vi "ConvertFormatElementsToItemList.vi"(11 "Format Elements":T1[](array[typedef])) -> (3 "Item List":string)   [LabVIEW 2012, in "Keithley-6485.lvlib"]
uses:
  Keithley-6485.lvlib
  Public/Controls/FormatElement.ctl
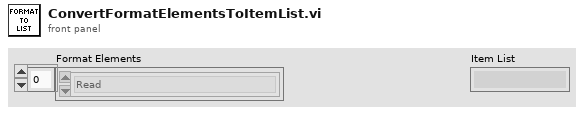
[diagram p1: front panel]
types:
  T1 = typedef "Keithley-6485.lvlib/FormatElement.ctl" = enum16{"Read", "Unit", "Time", "Status"}
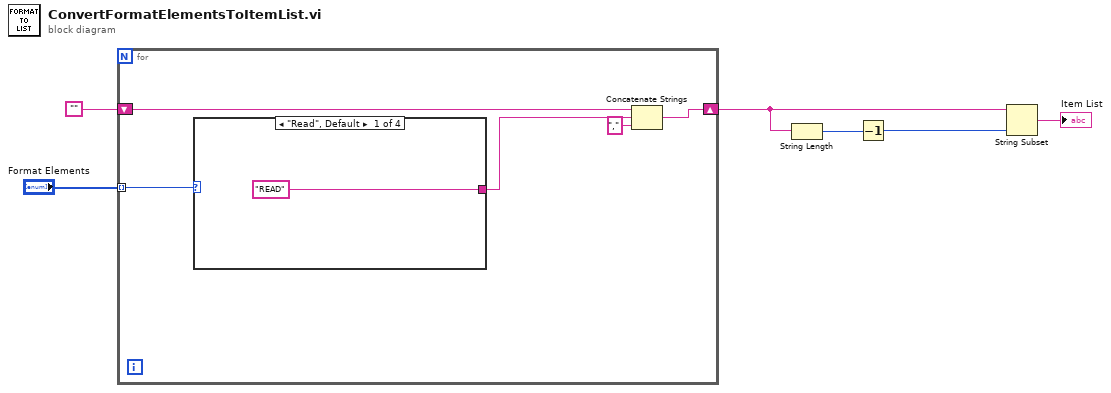
[diagram p0: block diagram]
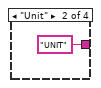
[diagram p2: hidden frame]
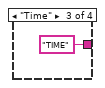
[diagram p3: hidden frame]
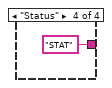
[diagram p4: hidden frame]
diagram:
  n1 = for {
    tunnel: "Format Elements" -> [w9] mode=indexing
    shift-right: [w10] -> w4
    shift-left: "" -> [w11]
    n2 = case shown="\"Read\", Default" w9 {
      tunnel: ["READ" "UNIT" "TIME" "STAT"] -> w8
      frame "Read", Default {
      }
      frame "Unit" {
      }
      frame "Time" {
      }
      frame "Status" {
      }
    }
    n3 = Concatenate Strings(w11, w8, "," ("string")) -> (w10:string)
  }
  n4 = String Length(string=w4) -> (length=w3:i32)
  n5 = Decrement(x=w3) -> (x-1=w2:i32)
  n6 = String Subset(string=w4, length (rest)=w2) -> (substring=→"Item List":string)  [unwired: 1 in]
